vi "SET_ActiveLayer.vi"(7 "Combine User Layers?":bool, 8 "error in (no error)":errorcluster, 10 "Layer.lvclass":refnum<class "Layer.lvclass">, 11 "Icon.lvclass in":refnum<class "Icon.lvclass">) -> (0 "error out":errorcluster, 3 "Icon.lvclass out":refnum<class "Icon.lvclass">)   [LabVIEW 2017, in "Icon.lvclass"]
doc: "Updates the currently active User Layer. Combine User Layers leaves the user the choice to merge all User Layers into one."
uses:
  <vilib>/LabVIEW Icon API/lv_icon/Classes/Icon/Icon.lvclass
  <vilib>/LabVIEW Icon API/lv_icon/Classes/Layer/Layer.lvclass
  <vilib>/LabVIEW Icon API/lv_icon/Classes/Icon/Icon.lvclass/Icon.ctl
  <vilib>/LabVIEW Icon API/lv_icon/Controls/Layer.ctl
  <vilib>/LabVIEW Icon API/lv_icon/lv_icon.lvlib
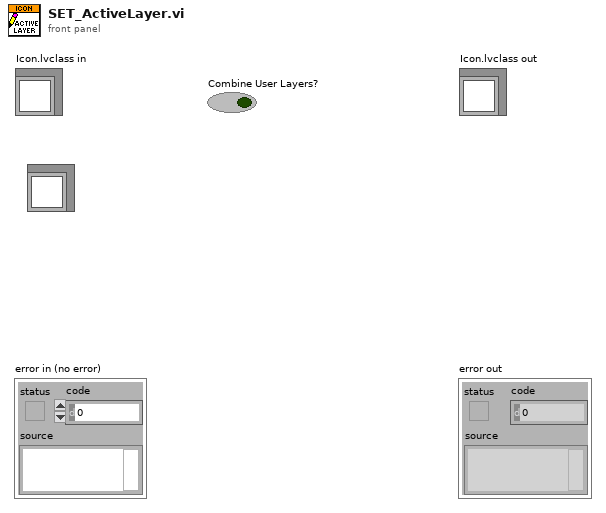
[diagram p1: front panel]
types:
  T1 = typedef "Layer.ctl" = cluster{"LayerIcon":picture, "LayerName":string, "Opacity":u8, "Visibility?":bool}
  T2 = typedef "LVPoint32TypeDef.ctl" = cluster{"Horizontal":i32, "Vertical":i32}
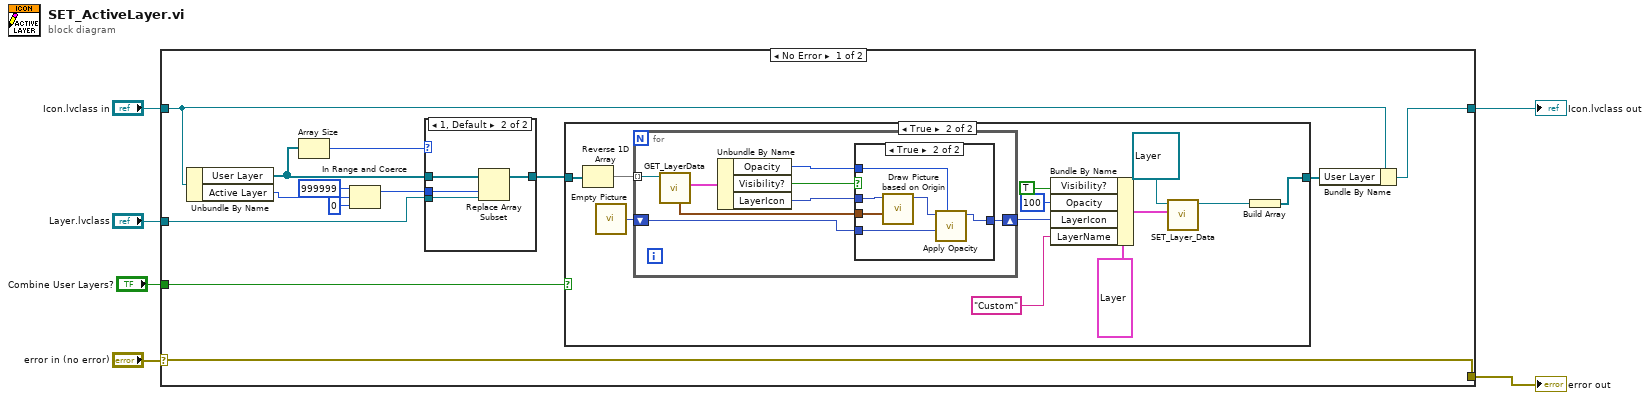
[diagram p0: block diagram]
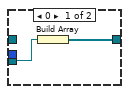
[diagram p4: hidden frame]
diagram:
  n1 = case shown="No Error" "error in (no error)" {
    selector: "error in (no error)" -> [w14 w54]
    tunnel: [w14 w54] -> w5
    tunnel: [w19 w55] -> w3
    tunnel: "Icon.lvclass in" -> [w18 w55]
    tunnel: "Layer.lvclass" -> [w17 _]
    tunnel: "Combine User Layers?" -> [w7 _]
    frame No Error {
      n2 = Unbundle By Name(w18) -> ("User Layer"=w16:refnum<class "Layer.lvclass">[], "Active Layer"=w9:i32)
      n3 = Array Size(array=w16) -> (size(s)=w15:i32)
      n4 = In Range and Coerce(upper limit=999999, x=w9, lower limit=0) -> (coerced(x)=w8:i32)  [unwired: 1 out]
      n5 = case shown="1, Default" w15 {
        tunnel: [w49 w53] -> w13
        tunnel: w17 -> [w48 w52]
        tunnel: w16 -> [_ w51]
        tunnel: w8 -> [_ w50]
        frame 0 {
          n6 = Build Array(w48) -> (w49:refnum<class "Layer.lvclass">[])
        }
        frame 1, Default {
          n7 = Replace Array Subset(array=w51, new element=w52, index=w50) -> (w53:refnum<class "Layer.lvclass">[])
        }
      }
      n8 = case shown="True" w7 {
        tunnel: w13 -> [w20 w23]
        tunnel: [w20 w22] -> w12
        frame False {
        }
        frame True {
          n9 = Reverse 1D Array(array=w23) -> (reversed array=w29:refnum<class "Layer.lvclass">[])
          n10 = call "Empty Picture"() -> ("empty picture"=w30:picture)
          n11 = for {
            shift-right: [w37] -> w26
            shift-left: w30 -> [w38]
            tunnel: w29 -> [w33] mode=indexing
            n12 = call-dynamic "GET_LayerData.vi"("Layer.lvclass in"=w33) -> ("Data"=w35:T1, "Origin"=w34:T2)  [unwired: 1 in, 8 out]
            n13 = Unbundle By Name(w35) -> ("Opacity"=w39:u8, "Visibility?"=w40:bool, "LayerIcon"=w36:picture)
            n14 = case shown="True" w40 {
              tunnel: w39 -> [_ w47]
              tunnel: w38 -> [w41 w46]
              tunnel: [w41 w45] -> w37
              tunnel: w36 -> [_ w44]
              tunnel: w34 -> [_ w43]
              frame False {
              }
              frame True {
                n15 = call <vilib>:"Draw Picture based on Origin.vi"("Origin"=w43, "LayerIcon in"=w44) -> ("LayerIcon out"=w42:picture)  [unwired: 1 in, 8 out]
                n16 = call <vilib>:"Apply Opacity.vi"("% (100)"=w47, "Bottom"=w46, "Top"=w42) -> ("new picture"=w45:picture)  [unwired: 8 out]
              }
            }
          }
          n17 = Bundle By Name(cluster=T1 {"LayerIcon"=bytes[0], "LayerName"="", "Opacity"=0, "Visibility?"=FALSE} ("Data"), "Visibility?"=TRUE, "Opacity"=u8 100, "LayerIcon"=w26, "LayerName"="Custom") -> (w27:T1)
          n18 = call-dynamic "SET_Layer_Data.vi"("Data"=w27, "Layer.lvclass in"=refnum<class "Layer.lvclass"> refnum) -> ("Layer.lvclass out"=w24:refnum<class "Layer.lvclass">)  [unwired: 2 in, 7 out]
          n19 = Build Array(w24) -> (w22:refnum<class "Layer.lvclass">[])
        }
      }
      n20 = Bundle By Name(cluster=w18, "User Layer"=w12) -> (w19:refnum<class "Icon.lvclass">)
    }
    frame Error {
    }
  }
  "error out" <- w5
  "Icon.lvclass out" <- w3
